vi "Filter.vi"(1 "In":dbl, 2 "Window":dbl=100.0 format="%#_13g") -> (0 "Out":dbl)   [LabVIEW 2014]
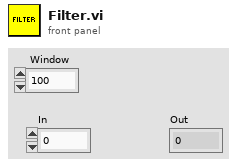
[diagram p1: front panel]
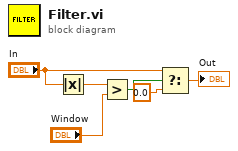
[diagram p0: block diagram]
diagram:
  n1 = Absolute Value(x="In") -> (abs(x)=w6:dbl)
  n2 = Greater?(x=w6, y="Window") -> (0:w5:bool)
  n3 = Select(t="In", s=w5, f=0.0) -> (s? t:f=→"Out":dbl)
